vi "Narvaez_Rommel-Erik_Carvajal-Labview.vi"() -> ()   [LabVIEW 2025]
uses:
  <vilib>/express/express arith-compare/Formula/XNode/ExpressFormulaBlockNode.xnode
panel:
  in  "Temperatura":dbl(slide) scale=-100.0..500.0
  out "Frio":bool
  out "Caliente":bool
  out "°C":dbl(knob) scale=-100.0..500.0
  out "°C":dbl(slide) scale=-100.0..500.0
  out "Celsius":dbl
  in  "STOP":bool
  out "°K":dbl(knob) scale=173.0..773.0
  out "°F":dbl(knob) scale=-148.0..932.0
  out "Kelvin":dbl
  out "Fahrenheit":dbl
  out "°K":dbl(slide) scale=173.0..773.0
  out "°F":dbl(slide) scale=-148.0..932.0
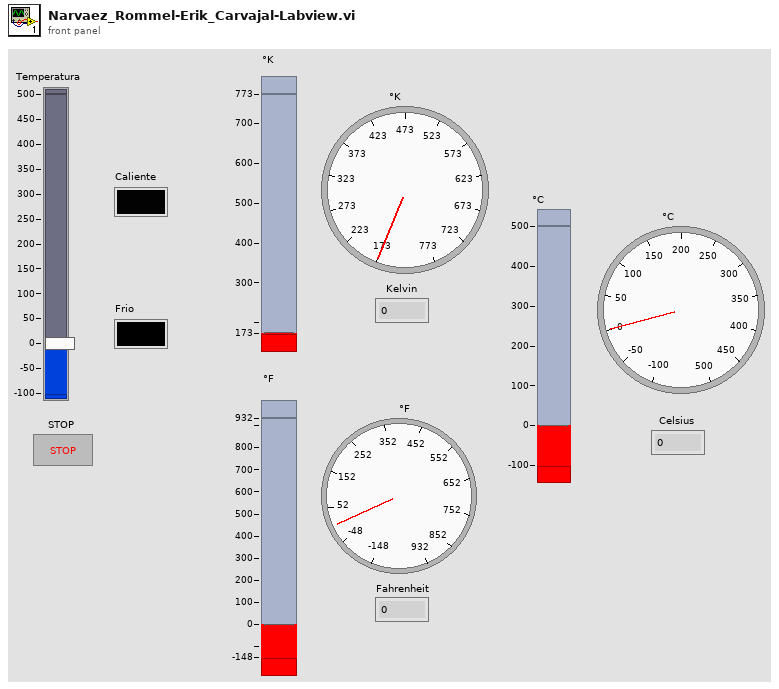
[diagram p1: front panel]
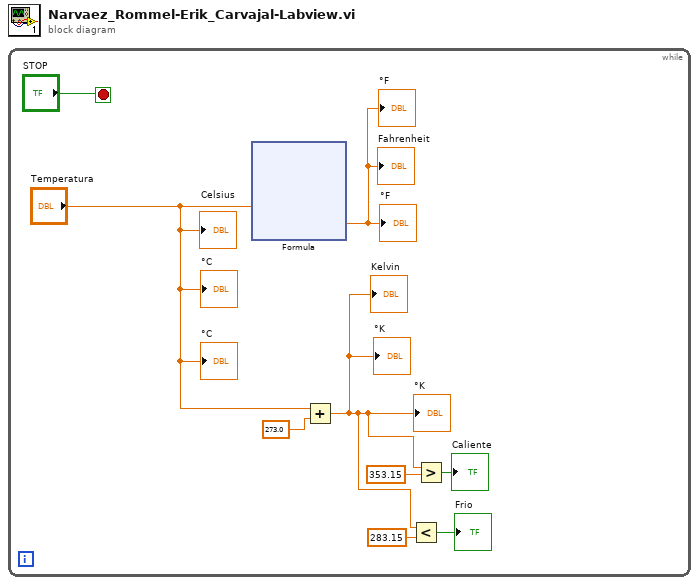
[diagram p0: block diagram]
diagram:
  n1 = while {
    stop <- "STOP" stop-if-true
    n2 = xnode "Formula"("X1"="Temperatura") -> ("Result"=→"°F" →"Fahrenheit" →"°F":dbl)  [unwired: 1 in, 1 out]
    n3 = Add(x="Temperatura", y=273.0) -> (x+y=w1:dbl)
    "°K" <- w1
    "Kelvin" <- w1
    "°K" <- w1
    n4 = Less?(x=w1, y=283.15) -> (x < y?=→"Frio":bool)
    n5 = Greater?(x=w1, y=353.15 ("x")) -> (0:→"Caliente":bool)
    "Celsius" <- "Temperatura"
    "°C" <- "Temperatura"
    "°C" <- "Temperatura"
  }
